vi "Start Chassis.vi"(5 "Cfg wChassis":T1, 6 "Show FP?":bool, 7 "Actor-to-Caller Enqueuer":refnum<class "Message Enqueuer.lvclass">, 8 "error in (no error)":errorcluster, 9 "TCP LS Writer":refnum<class "Message Enqueuer.lvclass">, 10 "TCP HS Writer":refnum<class "Message Enqueuer.lvclass">, 11 "Chassis Tasks in":refnum<class "Chassis Tasks.lvclass">) -> (0 "error out":errorcluster, 3 "Chassis Tasks out":refnum<class "Chassis Tasks.lvclass">)   [LabVIEW 2018, in "Data Acquisition.lvlib" / "Chassis Tasks.lvclass"]
uses:
  Chassis Tasks.lvclass
  <vilib>/ActorFramework/Message Enqueuer/Message Enqueuer.lvclass
  Custom Ctrls/Master Cfg/ge_Cfg wChassis.ctl
  Cfg Grandmaster/Class Chassis BOM/Chassis BOM.lvclass
  Cfg Grandmaster/Class Chassis Cfg/ChassisCfg.lvclass
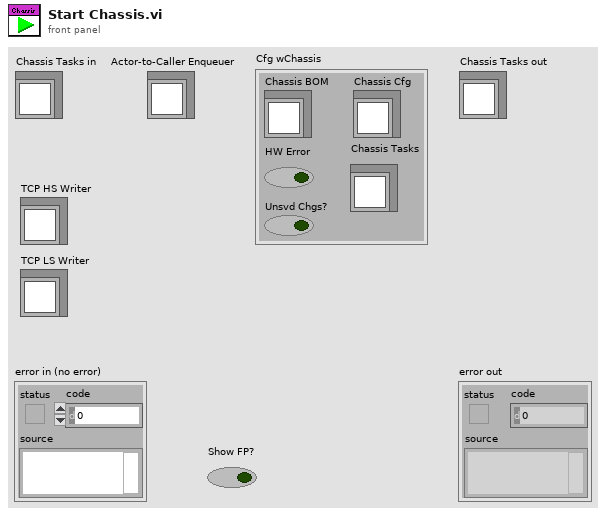
[diagram p1: front panel]
types:
  T1 = typedef "ge_Cfg wChassis.ctl" = cluster{"Chassis BOM":refnum<class "Chassis BOM.lvclass">, "Chassis Cfg":refnum<class "ChassisCfg.lvclass">, "Chassis Tasks":refnum<class "Chassis Tasks.lvclass">, "HW Error":bool, "Unsvd Chgs?":bool}
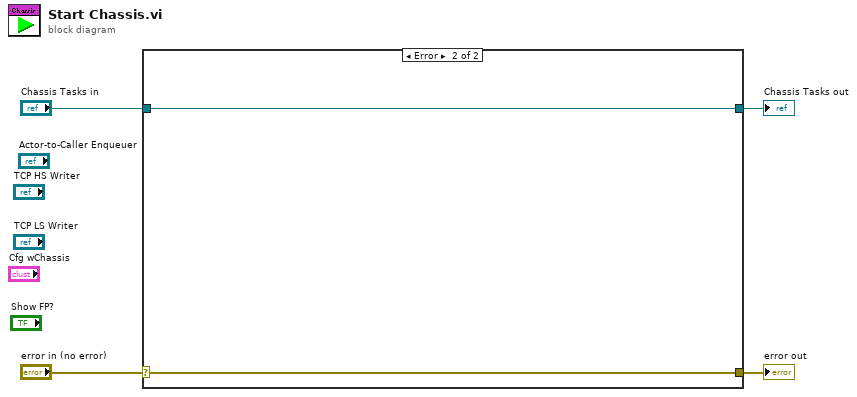
[diagram p0: block diagram]
diagram:
  n1 = case shown="Error" "error in (no error)" {
    selector: "error in (no error)" -> [w5 w8]
    tunnel: [w5 w8] -> w3
    tunnel: [w6 w7] -> w1
    tunnel: "Chassis Tasks in" -> [w6 w7]
    frame No Error {
      # "Wire the error cluster across even in the \"No Error\"\ncase so that warnings get propagated."
    }
    frame Error {
    }
  }
  "error out" <- w3
  "Chassis Tasks out" <- w1
